vi "Verify Grippee.vi"(8 "picture":picture) -> (0 "picture":picture, 3 "% match":dbl)   [LabVIEW 2013]
uses:
  <vilib>/Utility/file.llb/Read From Spreadsheet File (I64).vi
panel:
  out "points":i32
  out "Model":i64[][](graph)
  out "total":i32
  in  "file":path=path "C:/Program Files/Labview/user.lib/ROSforLV_0.1/Devices/Baxter/Cartesian/Grippee.csv"
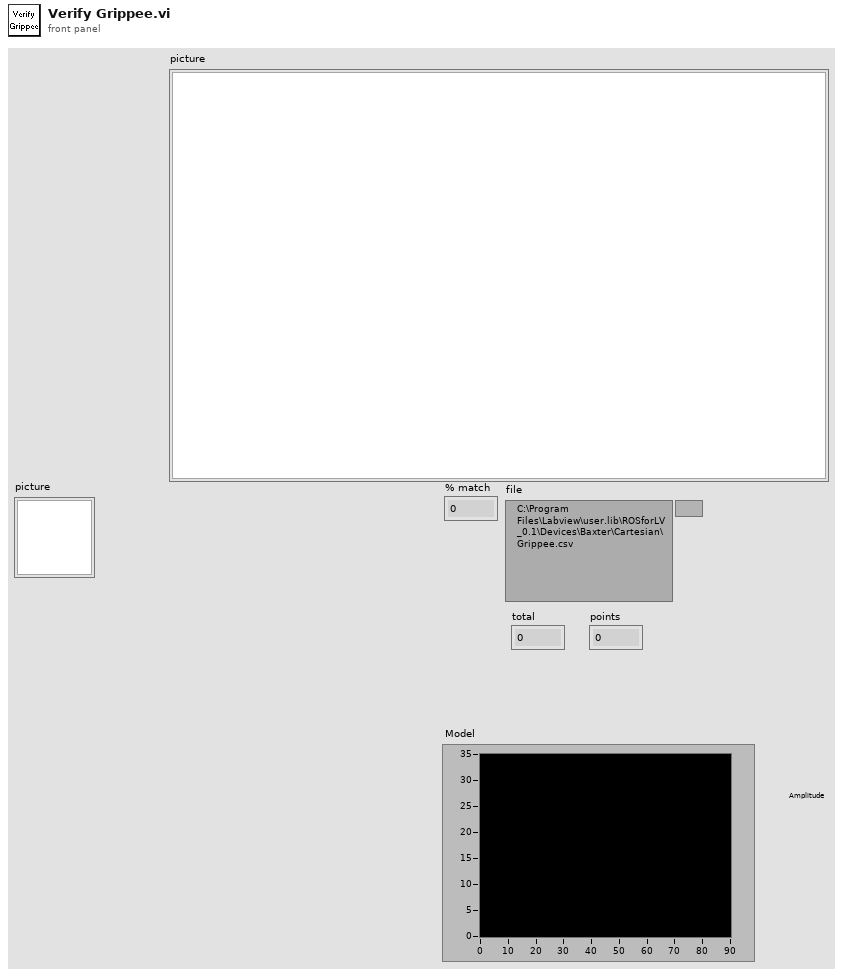
[diagram p1: front panel]
types:
  T1 = typedef "imagedata.ctl" = cluster{"image type":i32, "image depth":i32, "image":u8[], "mask":u8[], "colors":u32[], "Rectangle":cluster{"left":i16, "top":i16, "right":i16, "bottom":i16}}
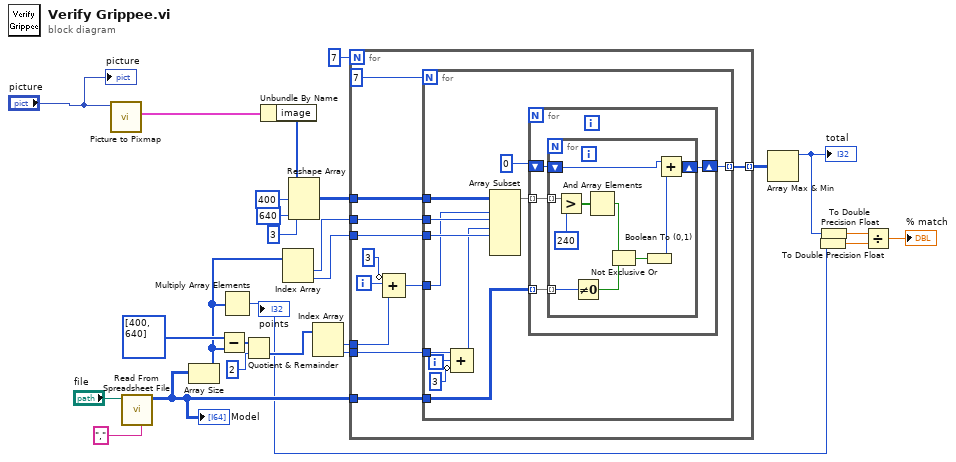
[diagram p0: block diagram]
diagram:
  n1 = call <vilib>:"Picture to Pixmap.vi"("picture"="picture") -> ("image data"=w15:T1)  [unwired: 9 in, 1 out]
  n2 = call-poly <vilib>:"Read From Spreadsheet File.vi"("delimiter (\\t)"="," ("delimiter (\\t)"), "file path (dialog if empty)"="file") -> ("all rows"=w12:i64[][])  [unwired: 5 in, 4 out]
  "Model" <- w12
  n3 = Array Size(array=w12) -> (size(s)=w13:i32[])
  n4 = Subtract(x=i32[] [400, 640], y=w13) -> (x-y=w20:i32[])
  n5 = Multiply Array Elements(1:w13) -> (0:w5:i32)
  "points" <- w5
  n6 = Quotient & Remainder(x=w20, y=2) -> (floor(x/y)=w9:i32[])  [unwired: 1 out]
  n7 = Unbundle By Name(w15) -> ("image"=w23:u8[])
  n8 = Index Array(array=w13) -> (element #1=w17:i32, element #2=w16:i32)  [unwired: 2 in]
  n9 = Reshape Array(w23, 400 ("dimension size"), 640 ("dimension size"), 3 ("dimension size")) -> (w18:u8[][][])
  n10 = Index Array(array=w9) -> (element #1=w8:i32, element #2=w7:i32)  [unwired: 2 in]
  n11 = for {
    N: 7 -> [_]
    tunnel: w18 -> [w37]
    tunnel: w17 -> [w36]
    tunnel: w16 -> [w35]
    tunnel: w12 -> [w34]
    tunnel: [w33] -> w11 mode=indexing
    tunnel: w8 -> [w29]
    tunnel: w7 -> [w27]
    i -> [w31]
    n12 = Compound Arithmetic op=ADD(invert 3 ("value"), w31, w29) -> (w28:i32)
    n13 = for {
      N: 7 -> [_]
      tunnel: w37 -> [w49]
      tunnel: w36 -> [w48]
      tunnel: w35 -> [w47]
      tunnel: w34 -> [w44]
      tunnel: [w43] -> w33 mode=indexing
      tunnel: w28 -> [w42]
      tunnel: w27 -> [w41]
      i -> [w40]
      n14 = Compound Arithmetic op=ADD(w41, w40, invert 3 ("value")) -> (w39:i32)
      n15 = Array Subset(array=w49, index (dim 0)=w42, length (dim 0)=w48, index (dim 1)=w39, length (dim 1)=w47) -> (w46:u8[][][])  [unwired: 2 in]
      n16 = for {
        tunnel: w46 -> [w53] mode=indexing
        tunnel: w44 -> [w52] mode=indexing
        shift-right: [w50] -> w43
        shift-left: 0 -> [w51]
        n17 = for {
          tunnel: w53 -> [w62] mode=indexing
          tunnel: w52 -> [w61] mode=indexing
          shift-right: [w60] -> w50
          shift-left: w51 -> [w59]
          n18 = Greater?(x=w62, y=u8 240) -> (0:w54:bool[])
          n19 = Not Equal To 0?(x=w61) -> (x != 0?=w55:bool)
          n20 = And Array Elements(Boolean array=w54) -> (logical AND=w56:bool)
          n21 = Not Exclusive Or(1:w55, 2:w56) -> (0:w57:bool)
          n22 = Boolean To (0,1)(Boolean=w57) -> (0, 1=w58:i16)
          n23 = Add(x=w59, y=w58) -> (x+y=w60:i32)
        }
      }
    }
  }
  n24 = Array Max & Min(array=w11) -> (max value=w6:i32)  [unwired: 3 out]
  "total" <- w6
  n25 = To Double Precision Float(number=w5) -> (double precision float=w3:dbl)
  n26 = To Double Precision Float(number=w6) -> (double precision float=w4:dbl)
  n27 = Divide(x=w4, y=w3) -> (x/y=→"% match":dbl)
  "picture" <- "picture"
